vi "PixyAverageX.vi"(11 "Input":dbl) -> (3 "mean":dbl)   [LabVIEW 2016]
uses:
  <vilib>/Analysis/baseanly.llb/Mean (DBL).vi
  <vilib>/Analysis/NI_AALBase.lvlib
panel:
  out "Past Array Out":dbl[](array[numeric])
  in  "Past Array":dbl[](array[numeric])
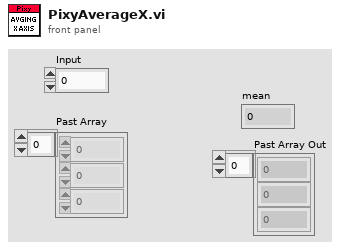
[diagram p1: front panel]
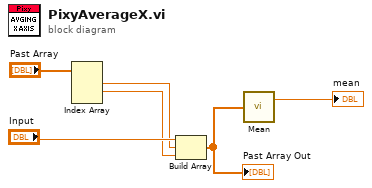
[diagram p0: block diagram]
diagram:
  n1 = Index Array(array="Past Array") -> (element #1=w4:dbl, element #2=w3:dbl)  [unwired: 3 in, 1 out]
  n2 = Build Array("Input", w4, w3) -> (w2:dbl[])
  "Past Array Out" <- w2
  n3 = call-poly <vilib>:"Mean.vi"("X"=w2) -> ("mean"=→"mean":dbl)  [unwired: 1 out]
